vi "fgv.vi"(7 "Command":T1, 9 "Name":string, 10 "DebugTracer":refnum<class "DebugTraceHandle.lvclass">) -> (0 "Remove/Found":bool, 1 "Array":refnum<class "DebugTraceHandle.lvclass">[](array[class]), 2 "DebugTracerOut":refnum<class "DebugTraceHandle.lvclass">)   [LabVIEW 2024, in "DebugTraceSingleton.lvlib"]
uses:
  DebugTraceSingleton.lvlib
  DebugTraceHandle/DebugTraceHandle.lvclass
  Command.ctl
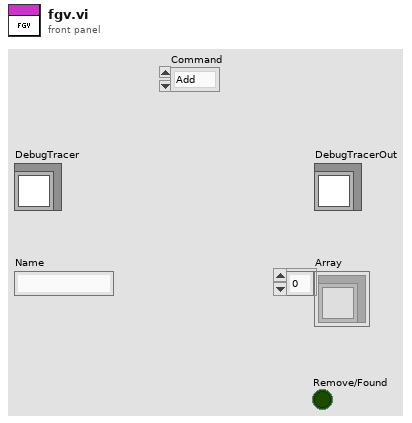
[diagram p1: front panel]
types:
  T1 = typedef "DebugTraceSingleton.lvlib/Command.ctl" = enum16{"Add", "Remove", "Get", "GetAll"}
  T2 = map{string, refnum<class "DebugTraceHandle.lvclass">}
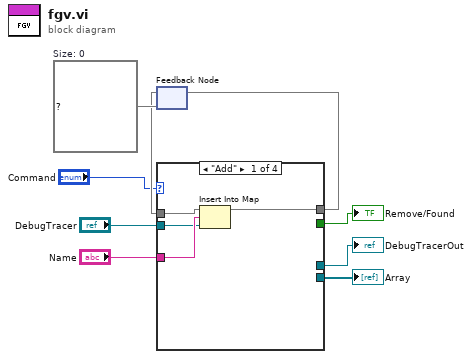
[diagram p0: block diagram]
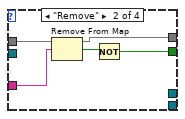
[diagram p2: hidden frame]
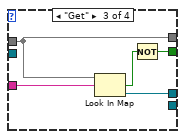
[diagram p3: hidden frame]
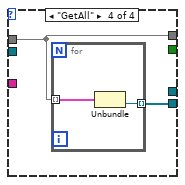
[diagram p4: hidden frame]
diagram:
  w9 = T2 {}  # Size: 0
  n1 = feedback #1(w9) -> (w8:T2)
  n2 = case shown="\"Add\"" "Command" {
    tunnel: w8 -> [w13 w18 w19 w24]
    tunnel: [w12 w17 w19 w24] -> w6
    tunnel: "Name" -> [w11 w16 w23 _]
    tunnel: "DebugTracer" -> [w10 _ _ _]
    tunnel: [_ w14 w20 _] -> w3
    tunnel: [_ _ w21 _] -> w2
    tunnel: [_ _ _ w25] -> w1
    frame "Add" {
      n3 = Insert Into Map(map in=w13, key=w11, value=w10) -> (map out=w12:T2)  [unwired: 2 out]
    }
    frame "Remove" {
      n4 = Remove From Map(10:w16, 11:w18) -> (2:w15:bool, 3:w17:T2)  [unwired: 1 out]
      n5 = Not(x=w15) -> (.not. x?=w14:bool)
    }
    frame "Get" {
      n6 = Look In Map(map=w19, key=w23) -> (key not found?=w22:bool, value=w21:refnum<class "DebugTraceHandle.lvclass">)  [unwired: 1 in]
      n7 = Not(x=w22) -> (.not. x?=w20:bool)
    }
    frame "GetAll" {
      n8 = for {
        tunnel: w24 -> [w27] mode=indexing
        tunnel: [w26] -> w25 mode=indexing
        n9 = Unbundle(w27) -> ("DebugTrace.lvlib:DebugTraceHandle.lvclass"=w26:refnum<class "DebugTraceHandle.lvclass">)  [unwired: 1 out]
      }
    }
  }
  "Remove/Found" <- w3
  "DebugTracerOut" <- w2
  "Array" <- w1
  n10 = feedback-in #1(w6) -> ()
